vi "Read Data DVR.vi"(8 "error in (no error)":errorcluster, 11 "nPAS in":refnum<class "nPAS.lvclass">) -> (0 "error out":errorcluster, 2 "Data DVR":refnum<data-value>, 3 "nPAS out":refnum<class "nPAS.lvclass">)   [LabVIEW 2016, in "gPAS Library.lvlib" / "nPAS.lvclass"]
uses:
  nPAS.lvclass
  Data/SOAP Data.lvclass
  nPAS.lvclass/nPAS.ctl
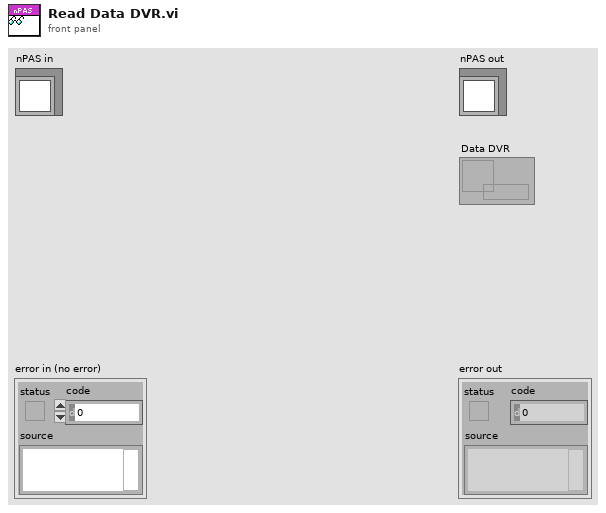
[diagram p1: front panel]
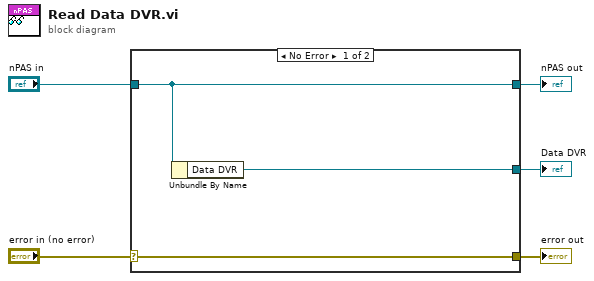
[diagram p0: block diagram]
diagram:
  n1 = case shown="No Error" "error in (no error)" {
    selector: "error in (no error)" -> [w8 w9]
    tunnel: [w8 w9] -> w4
    tunnel: [w7 w10] -> w2
    tunnel: "nPAS in" -> [w7 w10]
    tunnel: [w6 _] -> w1
    frame No Error {
      n2 = Unbundle By Name(w7) -> ("Data DVR"=w6:refnum<data-value>)
    }
    frame Error {
    }
  }
  "error out" <- w4
  "nPAS out" <- w2
  "Data DVR" <- w1
